vi "给选中单元格上色.vi"(6 "颜色":cluster{"未选中颜色盒":u32, "选中颜色盒":u32}={"未选中颜色盒"=16763272, "选中颜色盒"=12439011}, 8 "错误输入（无错误）":errorcluster, 9 "本次坐标":T1={"Row"=20, "Column"=20}, 10 "上次坐标":T1={"Row"=20, "Column"=20}, 11 "引用输入":refnum<vi>) -> (0 "错误输出":errorcluster, 2 "上次坐标输出":T1={"Row"=20, "Column"=20}, 3 "引用输出":refnum<vi>)   [LabVIEW 2014, in "表格.lvlib" / "表格上色.lvlib"]
uses:
  <vilib>/Utility/miscctls.llb/LVRowAndColumnTypeDef.ctl
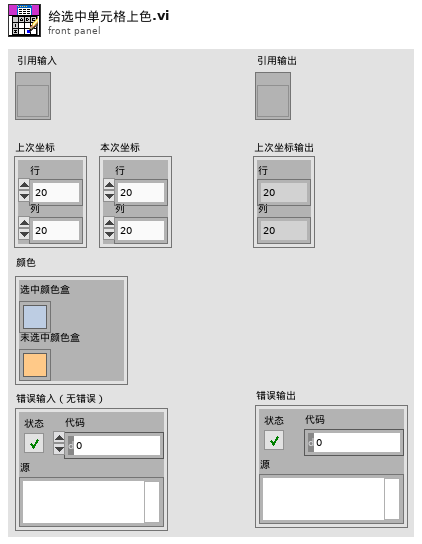
[diagram p1: front panel]
types:
  T1 = typedef "LVRowAndColumnTypeDef.ctl" = cluster{"Row":i32, "Column":i32}
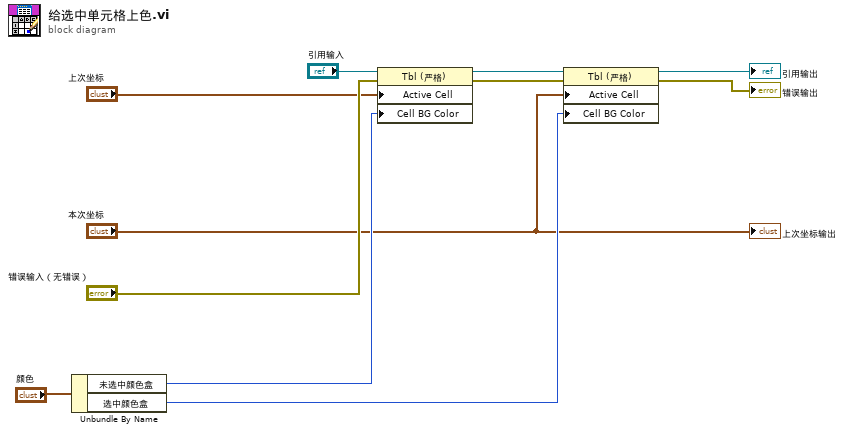
[diagram p0: block diagram]
diagram:
  n1 = Unbundle By Name("颜色") -> ("未选中颜色盒"=w10:u32, "选中颜色盒"=w9:u32)
  n2 = property on="属性节点" class="Tbl (严格)"(reference="引用输入", error in="错误输入（无错误）", "Active Cell"="上次坐标", "Cell BG Color"=w10) -> (reference out=w3:refnum<vi>, error out=w2:errorcluster)
  n3 = property on="属性节点" class="Tbl (严格)"(reference=w3, error in=w2, "Active Cell"="本次坐标", "Cell BG Color"=w9) -> (reference out=→"引用输出":refnum<vi>, error out=→"错误输出":errorcluster)
  "上次坐标输出" <- "本次坐标"
